vi "Load from INI from Refs.vi"(10 "Configuration file path":path, 11 "Array of Control References":refnum<vi>[](array[refnum])) -> ()   [LabVIEW 2019]
uses:
  <vilib>/Utility/config.llb/Read Key (Path).vi
  <vilib>/Utility/config.llb/Read Key (Boolean).vi
  <vilib>/Utility/config.llb/Read Key (Double).vi
  <vilib>/Utility/config.llb/Read Key (String).vi
  <vilib>/Utility/config.llb/Read Key (I32).vi
  <vilib>/Utility/config.llb/Read Key (U32).vi
  <vilib>/Utility/config.llb/NI_LVConfig.lvlib
panel:
  out "Control Types Array":string[](array[string])
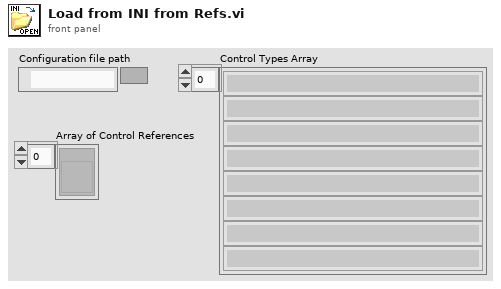
[diagram p1: front panel]
types:
  T1 = typedef "NI_LVConfig.lvlib/Config Data RefNum.ctl" = refnum<k1>
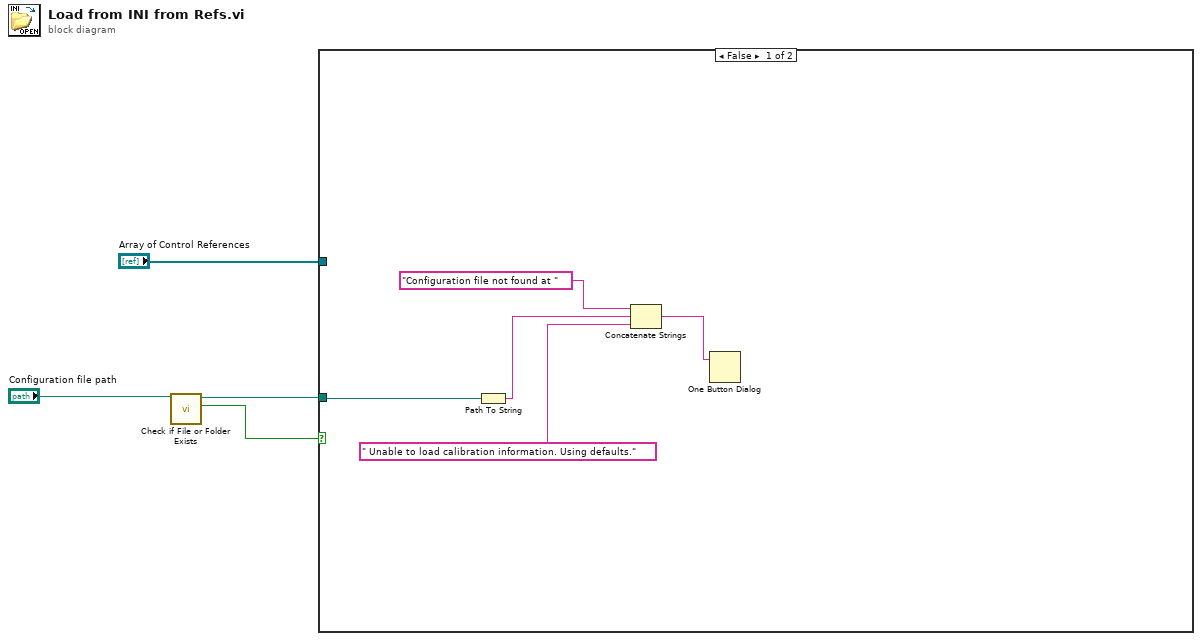
[diagram p0: block diagram]
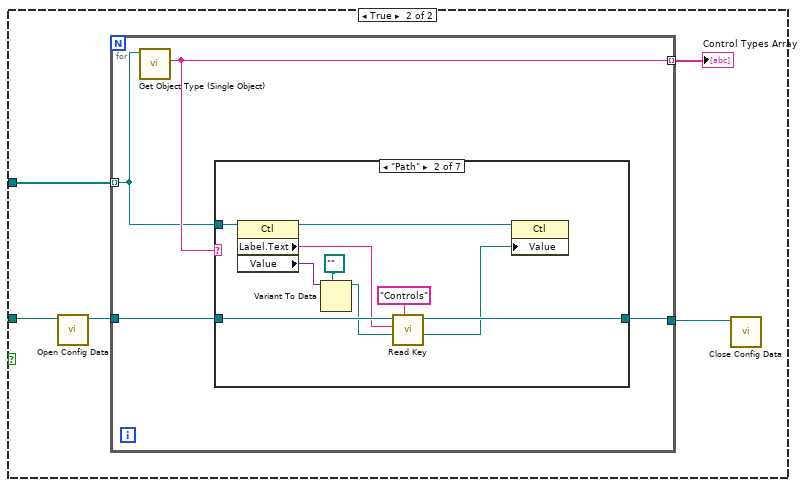
[diagram p2: hidden frame]
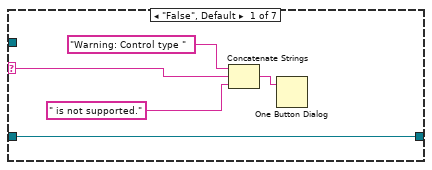
[diagram p3: hidden frame]
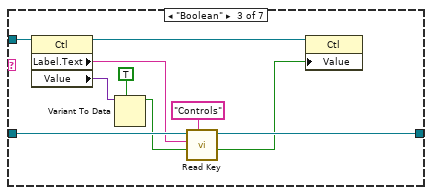
[diagram p4: hidden frame]
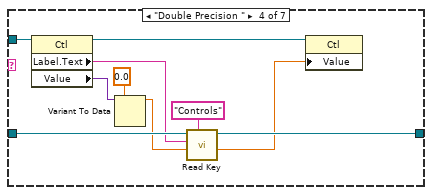
[diagram p5: hidden frame]
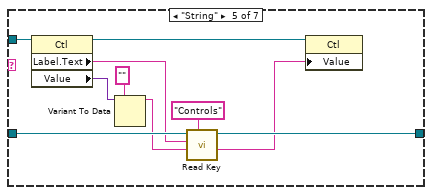
[diagram p6: hidden frame]
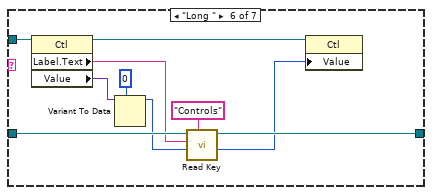
[diagram p7: hidden frame]
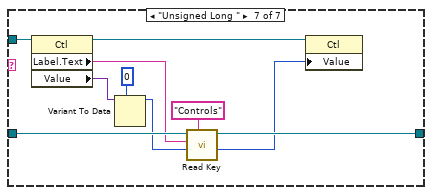
[diagram p8: hidden frame]
diagram:
  n1 = call <vilib>:"Check if File or Folder Exists.vi"("path"="Configuration file path") -> ("file or folder exists?"=w1:bool, "dup path"=w2:path)  [unwired: 8 in, 1 out]
  n2 = case shown="False" w1 {
    tunnel: "Array of Control References" -> [_ w14]
    tunnel: w2 -> [w8 w10]
    frame False {
      n3 = Path To String(path=w8) -> (string=w7:string)
      n4 = Concatenate Strings("Configuration file not found at " ("string"), w7, " Unable to load calibration information. Using defaults." ("string")) -> (w6:string)
      n5 = One Button Dialog(message=w6) -> ()  [unwired: 1 in, 1 out]
    }
    frame True {
      n6 = call <vilib>:"Open Config Data.vi"("configuration file path"=w10) -> ("refnum"=w11:T1)  [unwired: 8 in, 2 out]
      n7 = for {
        tunnel: w14 -> [w15] mode=indexing
        tunnel: [w16] -> w13 mode=indexing
        tunnel: [w17] -> w12
        tunnel: w11 -> [w18]
        n8 = call "Get Object Type (Single Object).vi"("Object Reference"=w15) -> ("Object Type"=w16:string)  [unwired: 8 in, 2 out]
        n9 = case shown="\"Path\"" w16 {
          selector: w16 -> [w21 _ _ _ _ _ _]
          tunnel: w18 -> [w23 w31 w42 w52 w62 w72 w82]
          tunnel: [w23 w29 w40 w50 w60 w70 w80] -> w17
          tunnel: w15 -> [_ w32 w43 w53 w63 w73 w83]
          frame "False", Default {
            n10 = Concatenate Strings("Warning: Control type " ("string"), w21, " is not supported." ("string")) -> (w19:string)
            n11 = One Button Dialog(message=w19) -> ()  [unwired: 1 in, 1 out]
          }
          frame "Path" {
            n12 = property class="Ctl"(reference=w32) -> (reference out=w25:refnum<vi>, "Label.Text"=w28:string, "Value"=w27:variant)  [unwired: 1 in, 1 out]
            n13 = Variant To Data(type=path "", Variant=w27) -> (data=w26:path)  [unwired: 1 in, 1 out]
            n14 = call-poly <vilib>:"Read Key.vi"("section"="Controls", "default value"=w26, "key"=w28, "refnum"=w31) -> ("value"=w24:path, "refnum out"=w29:T1)  [unwired: 4 in, 2 out]
            n15 = property class="Ctl"(reference=w25, "Value"=w24) -> ()  [unwired: 1 in, 2 out]
          }
          frame "Boolean" {
            n16 = property class="Ctl"(reference=w43) -> (reference out=w36:refnum<vi>, "Label.Text"=w39:string, "Value"=w38:variant)  [unwired: 1 in, 1 out]
            n17 = Variant To Data(type=TRUE, Variant=w38) -> (data=w37:bool)  [unwired: 1 in, 1 out]
            n18 = call-poly <vilib>:"Read Key.vi"("section"="Controls", "default value"=w37, "key"=w39, "refnum"=w42) -> ("value"=w35:bool, "refnum out"=w40:T1)  [unwired: 4 in, 2 out]
            n19 = property class="Ctl"(reference=w36, "Value"=w35) -> ()  [unwired: 1 in, 2 out]
          }
          frame "Double Precision " {
            n20 = property class="Ctl"(reference=w53) -> (reference out=w46:refnum<vi>, "Label.Text"=w49:string, "Value"=w48:variant)  [unwired: 1 in, 1 out]
            n21 = Variant To Data(type=0.0, Variant=w48) -> (data=w47:dbl)  [unwired: 1 in, 1 out]
            n22 = call-poly <vilib>:"Read Key.vi"("section"="Controls", "default value"=w47, "key"=w49, "refnum"=w52) -> ("value"=w45:dbl, "refnum out"=w50:T1)  [unwired: 4 in, 2 out]
            n23 = property class="Ctl"(reference=w46, "Value"=w45) -> ()  [unwired: 1 in, 2 out]
          }
          frame "String" {
            n24 = property class="Ctl"(reference=w63) -> (reference out=w56:refnum<vi>, "Label.Text"=w59:string, "Value"=w58:variant)  [unwired: 1 in, 1 out]
            n25 = Variant To Data(type="", Variant=w58) -> (data=w57:string)  [unwired: 1 in, 1 out]
            n26 = call-poly <vilib>:"Read Key.vi"("section"="Controls", "default value"=w57, "key"=w59, "refnum"=w62) -> ("value"=w55:string, "refnum out"=w60:T1)  [unwired: 4 in, 2 out]
            n27 = property class="Ctl"(reference=w56, "Value"=w55) -> ()  [unwired: 1 in, 2 out]
          }
          frame "Long " {
            n28 = property class="Ctl"(reference=w73) -> (reference out=w66:refnum<vi>, "Label.Text"=w69:string, "Value"=w68:variant)  [unwired: 1 in, 1 out]
            n29 = Variant To Data(type=0 ("Integer - Long"), Variant=w68) -> (data=w67:i32)  [unwired: 1 in, 1 out]
            n30 = call-poly <vilib>:"Read Key.vi"("section"="Controls", "default value"=w67, "key"=w69, "refnum"=w72) -> ("value"=w65:i32, "refnum out"=w70:T1)  [unwired: 4 in, 2 out]
            n31 = property class="Ctl"(reference=w66, "Value"=w65) -> ()  [unwired: 1 in, 2 out]
          }
          frame "Unsigned Long " {
            n32 = property class="Ctl"(reference=w83) -> (reference out=w76:refnum<vi>, "Label.Text"=w79:string, "Value"=w78:variant)  [unwired: 1 in, 1 out]
            n33 = Variant To Data(type=u32 0 ("Integer - Unsigned Long"), Variant=w78) -> (data=w77:u32)  [unwired: 1 in, 1 out]
            n34 = call-poly <vilib>:"Read Key.vi"("section"="Controls", "default value"=w77, "key"=w79, "refnum"=w82) -> ("value"=w75:u32, "refnum out"=w80:T1)  [unwired: 4 in, 2 out]
            n35 = property class="Ctl"(reference=w76, "Value"=w75) -> ()  [unwired: 1 in, 2 out]
          }
        }
      }
      "Control Types Array" <- w13
      n36 = call <vilib>:"Close Config Data.vi"("refnum"=w12) -> ()  [unwired: 9 in, 2 out]
    }
  }
